vi "Test Buffer Control.vi"() -> ()   [LabVIEW 2016]
doc: "This VI provides an example of the use of an X-control that serves as a 2-D buffer. The X-control stores data as channel data and variable data. Any number of channels may be viewed using the X-control display for a single variable, but only one variable may be viewed at a time. \n\nThis control is most useful for storing and visualizing low frequency data (such as housekeeping data on a data acquisition system). Due to the nature of X-controls, this method is not ideal for storage of high frequency data (runs on the UI thread so it will cause issues with any interface)."
uses:
  2D Control/2D Buffer Display.xctl
  <vilib>/Platform/TimedLoop/XDataNode/timing_clust.ctl
  <vilib>/Platform/TimedLoop/XDataNode/nitl_modes.ctl
  <vilib>/Platform/TimedLoop/XDataNode/wakeup.ctl
  <vilib>/Platform/TimedLoop/XDataNode/XDataNode.xnode
  <vilib>/Platform/TimedLoop/XDataNode/XDNodeRunTimeDep.lvlib
panel:
  out "Avg Data":T1(array[cluster])
  in  "data":cluster{"dat 1":sgl, "dat 2":sgl}
  in  "stop":bool
  out "2d_buffer":cluster{"data_out":sgl[][], "time":timestamp}(xcontrol)
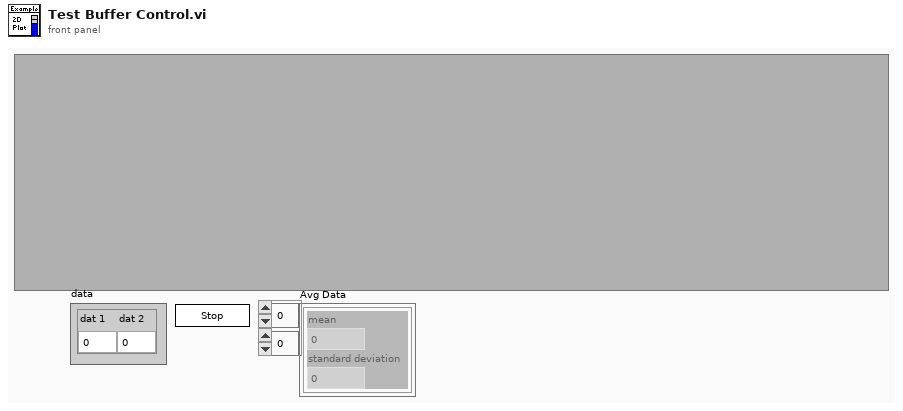
[diagram p1: front panel]
types:
  T1 = cluster{"mean":dbl, "standard deviation":dbl}[][]
  T2 = cluster{"Name":string, "Line Width":u8, "Line Style":u8, "Color":u32}[]
  T3 = typedef "XDNodeRunTimeDep.lvlib/timing_clust.ctl" = cluster{"Expected End [f-1]":u64, "Actual End [f-1]":u64, "Finished Late? [f-1]":bool, "Expected End [i-1]":u64, "Actual End [i-1]":u64, "Finished Late? [i-1]":bool, "Expected Start [i]":u64, "Actual Start [i]":u64, "Expected Start [f]":u64, "Actual Start [f]":u64, "Source Name":string, "Structure Name":string, "Period":i64, "Deadline":i64, "Offset":i64, "Start":i64, "Priority":i32, "Timeout":i32, "Mode":T4, "Wakeup Reason":T5, "Error":errorcluster, "Source Type":string, "Secondary Source Type":string, "Global End Time":u64, "Global Start Time":u64, "Frame Duration":u64, "Iteration Duration":u64, "Assigned CPU":i32, "I/O Scan Engine Mode":u32}
  T4 = typedef "XDNodeRunTimeDep.lvlib/nitl_modes.ctl" = enum32{"No Change", "Process missed periods, maintain original phase", "Discard missed periods, maintain original phase", "Process missed periods, ignore original phase", "Discard missed periods, ignore original phase"}
  T5 = typedef "XDNodeRunTimeDep.lvlib/wakeup.ctl" = enum32{"Normal", "Aborted", "Asynchronous wakeup", "Timing source error", "Timed loop error", "Timeout"}
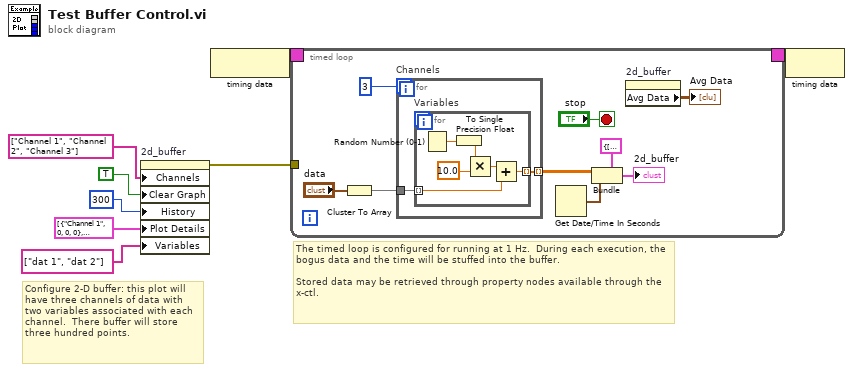
[diagram p0: block diagram]
diagram:
  # "The timed loop is configured for running at 1 Hz.  During each execution, the bogus data and the time will be stuffed into the buffer.\n\nStored data may be retrieved through property nodes available through the x-ctl."
  # "Configure 2-D buffer: this plot will have three channels of data with two variables associated with each channel.  There buffer will store three hundred points."
  n1 = property on="2d_buffer" class="2D Buffer Display (strict)"("Channels"=string[] ["Channel 1", "Channel 2", "Channel 3"], "Clear Graph"=TRUE, "History"=u16 300, "Plot Details"=T2 [{"Name"="Channel 1", "Line Width"=0, "Line Style"=0, "Color"=0}, {"Name"="Channel 2", "Line Width"=2, "Line Style"=1, "Color"=16711680}, {"Name"="Channel 2", "Line Width"=2, "Line Style"=0, "Color"=16860}], "Variables"=string[] ["dat 1", "dat 2"]) -> (error out=w5:errorcluster)  [unwired: 2 in, 1 out]
  n2 = node-c288() -> (w2:T3)
  n3 = timed-loop {
    tunnel: w5 -> [_]
    timing: w2 -> [_]
    timing-out: [_] -> w1
    stop <- "stop" stop-if-true
    n4 = Cluster To Array(cluster="data") -> (array=w10:sgl[])
    n5 = for "Channels" {
      N: 3 -> [_]
      tunnel: w10 -> [w19]
      tunnel: [w18] -> w14 mode=indexing
      n6 = for "Variables" {
        tunnel: w19 -> [w23] mode=indexing
        tunnel: [w22] -> w18 mode=indexing
        n7 = Random Number (0-1)() -> (number: 0 to 1=w21:dbl)
        n8 = To Single Precision Float(number=w21) -> (single precision float=w20:sgl)
        n9 = Multiply(x=w20, y=sgl 10.0) -> (x*y=w24:sgl)
        n10 = Add(x=w24, y=w23) -> (x+y=w22:sgl)
      }
    }
    n11 = Get Date/Time In Seconds() -> (seconds since 1Jan1904=w15:timestamp)
    n12 = Bundle(cluster=cluster{"data_out":sgl[][], "time":timestamp} {"data_out"=[], "time"=timestamp(0 s since 1904-01-01)} ("2D Buffer Display"), "data_out"=w14, "time"=w15) -> (→"2d_buffer":cluster{"data_out":sgl[][], "time":timestamp})
    n13 = property on="2d_buffer" class="2D Buffer Display (strict)"() -> ("Avg Data"=→"Avg Data":T1)  [unwired: 2 in, 2 out]
  }
  n14 = node-c288(w1) -> ()
